vi "tsdiag_can_security_access_request_seed.vi"(8 "ATimeoutMS":i32, 9 "ALevel":i32, 10 "ADiagModuleIndex":i32, 11 "路径输入":path) -> (1 "ARecSeed 2":u8[](array[numeric]), 2 "返回类型":i32, 3 "路径输出":path)   [LabVIEW 2019]
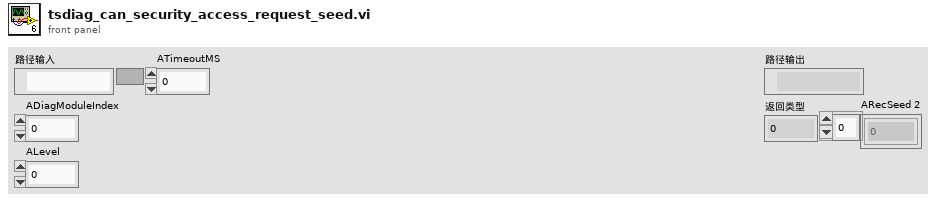
[diagram p1: front panel]
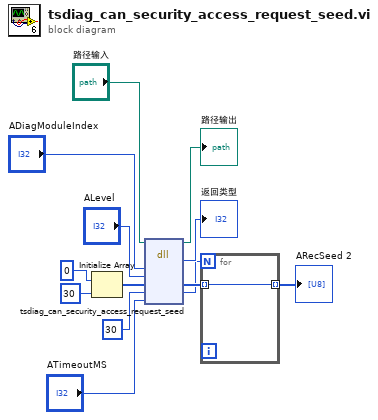
[diagram p0: block diagram]
diagram:
  n1 = Initialize Array(u8 0 ("元素"), 30 ("维数大小")) -> (w3:u8[])
  n2 = dll-call lib="C:/Users/XYY/Desktop/LabView Demo/TSCAN_LB2018_V1.4_20220309/Config/TSMaster.dll" fn="tsdiag_can_security_access_request_seed"(path in="路径输入", "ADiagModuleIndex"="ADiagModuleIndex", "ALevel"="ALevel", "ARecSeed"=w3, "ARecSeedSize"=30, "ATimeoutMS"="ATimeoutMS") -> (path out=→"路径输出":path, "返回类型"=→"返回类型":i32, "ARecSeed"=w7:u8[], "ARecSeedSize"=w6:i32)  [unwired: 5 in, 1 out]
  n3 = for {
    N: w6 -> [_]
    tunnel: w7 -> [w14] mode=indexing
    tunnel: [w14] -> w5 mode=indexing
  }
  "ARecSeed 2" <- w5
